vi "insert.vi"(8 "error in (no error)":errorcluster, 11 "DataCollectionDL110128Streaming in":refnum<class "DataCollectionDL110128Streaming.lvclass">) -> (0 "error out":errorcluster, 3 "DataCollectionDL110128Streaming out":refnum<class "DataCollectionDL110128Streaming.lvclass">)   [LabVIEW 2010, in "DataCollectionDL110128Streaming.lvclass"]
uses:
  DataCollectionDL110128Streaming.lvclass
  DataCollectionDL110128Streaming.lvclass/DataCollectionDL110128Streaming.ctl
  common/classes/GenericComponent/GenericComponent/class_data.vi
  common/classes/GenericComponent/GenericComponent/GenericComponent.lvclass
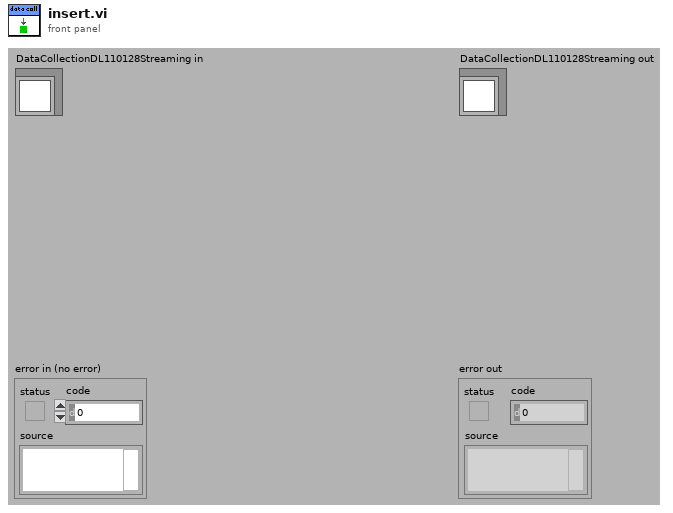
[diagram p1: front panel]
types:
  T1 = enum16{"open", "replace", "create", "open or create", "replace or create", "replace or create with confirmation"}
  T2 = typedef "pixel_raw_data_array.ctl" = dbl[][]
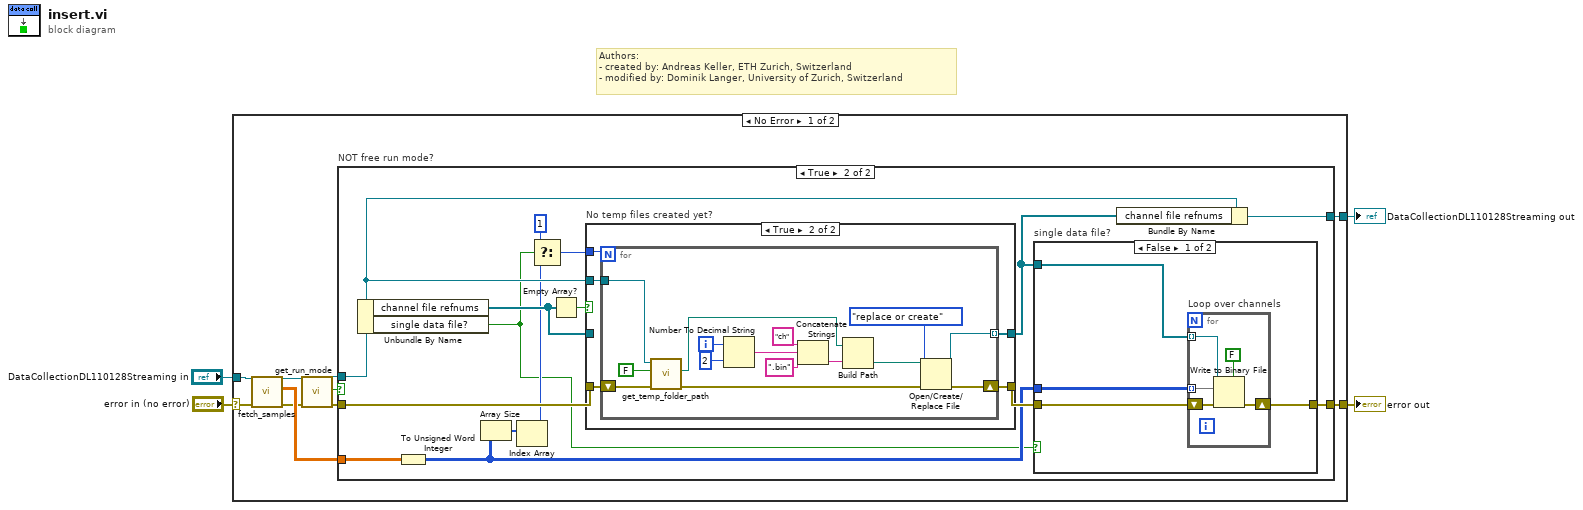
[diagram p0: block diagram]
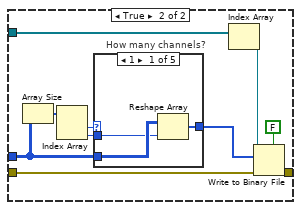
[diagram p3: hidden frame]
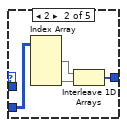
[diagram p4: hidden frame]
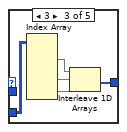
[diagram p5: hidden frame]
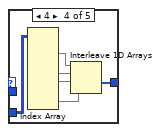
[diagram p6: hidden frame]
diagram:
  # "Authors: \n- created by: Andreas Keller, ETH Zurich, Switzerland\n- modified by: Dominik Langer, University of Zurich, Switzerland"
  n1 = case shown="No Error" "error in (no error)" {
    selector: "error in (no error)" -> [w13 w92]
    tunnel: [w12 w92] -> w3
    tunnel: [w11 w91] -> w1
    tunnel: "DataCollectionDL110128Streaming in" -> [w14 w91]
    frame No Error {
      n2 = call-dynamic "fetch_samples.vi"("error in (no error)"=w13, "GenericToplevelComponent in"=w14) -> ("error out"=w9:errorcluster, "channels raw data block"=w10:T2, "GenericToplevelComponent out"=w7:refnum<class "DataCollectionDL110128Streaming.lvclass">)  [unwired: 6 in, 1 out]
      n3 = call "get_run_mode.vi"("error in (no error)"=w9, "GenericPlugin in"=w7) -> ("error out"=w8:errorcluster, "GenericPlugin out"=w5:refnum<class "DataCollectionDL110128Streaming.lvclass">, "is NOT free run?"=w6:bool)  [unwired: 5 in, 2 out]
      n4 = case "NOT free run mode?" shown="True" w6 {
        tunnel: [w16 w29] -> w12
        tunnel: [w15 w27] -> w11
        tunnel: w10 -> [_ w23]
        tunnel: w8 -> [w16 w25]
        tunnel: w5 -> [w15 w24]
        frame False {
        }
        frame True {
          n5 = Unbundle By Name(w24) -> ("channel file refnums"=w31:refnum<file>[], "single data file?"=w17:bool)
          n6 = To Unsigned Word Integer(number=w23) -> (unsigned 16bit integer=w22:u16[][])
          n7 = Array Size(array=w22) -> (size(s)=w21:i32[])
          n8 = Index Array(array=w21) -> (element=w18:i32)  [unwired: 1 in]
          n9 = Select(t=1, s=w17, f=w18) -> (s? t:f=w20:i32)
          n10 = Empty Array?(array=w31) -> (empty?=w26:bool)
          n11 = case "No temp files created yet?" shown="True" w26 {
            tunnel: w25 -> [w70 w75]
            tunnel: [w70 w74] -> w30
            tunnel: w31 -> [w69 _]
            tunnel: [w69 w73] -> w28
            tunnel: w24 -> [_ w72]
            tunnel: w20 -> [_ w71]
            frame False {
            }
            frame True {
              n12 = for {
                N: w71 -> [_]
                shift-right: [w90] -> w74
                shift-left: w75 -> [w89]
                tunnel: [w88] -> w73 mode=indexing
                tunnel: w72 -> [w87]
                i -> [w83]
                n13 = call-dynamic "get_temp_folder_path.vi"("error in (no error)"=w89, "flush?"=FALSE, "GenericComponent in"=w87) -> ("error out"=w77:errorcluster, "temp path"=w76:path)  [unwired: 6 in, 1 out]
                n14 = Number To Decimal String(number=w83, width (-)=i16 2) -> (decimal integer string=w81:string)
                n15 = Concatenate Strings("ch", w81, ".bin") -> (w80:string)
                n16 = Build Path(base path=w76, name or relative path=w80) -> (appended path=w84:path)
                n17 = Open/Create/Replace File(file path (use dialog)=w84, error in=w77, operation (0:open)=T1."replace or create") -> (refnum out=w88:refnum<file>, error out=w90:errorcluster)  [unwired: 3 in, 1 out]
              }
            }
          }
          n18 = case "single data file?" shown="False" w17 {
            tunnel: w30 -> [w35 w47]
            tunnel: [w34 w46] -> w29
            tunnel: w28 -> [w33 w49]
            tunnel: w22 -> [w32 w41]
            frame False {
              n19 = for "Loop over channels" {
                tunnel: w33 -> [w38] mode=indexing
                tunnel: w32 -> [w36] mode=indexing
                shift-right: [w39] -> w34
                shift-left: w35 -> [w40]
                n20 = Write to Binary File(file (use dialog)=w38, data=w36, error in=w40, 5:FALSE ("prepend array or string size? (T)")) -> (error out=w39:errorcluster)  [unwired: 2 in, 2 out]
              }
            }
            frame True {
              n21 = Array Size(array=w41) -> (size(s)=w45:i32[])
              n22 = Index Array(array=w45) -> (element #1=w44:i32, element #2=w43:i32)  [unwired: 2 in]
              n23 = case "How many channels?" shown="1" w44 {
                tunnel: w41 -> [w53 w56 w60 w64 _]
                tunnel: w43 -> [w52 _ _ _ _]
                tunnel: [w51 w57 w59 w65 _] -> w42
                frame 1 {
                  n24 = Reshape Array(w53, w52) -> (w51:u16[])
                }
                frame 2 {
                  n25 = Index Array(array=w56) -> (element #1=w55:u16[], element #2=w54:u16[])  [unwired: 4 in]
                  n26 = Interleave 1D Arrays(w55, w54) -> (w57:u16[])
                }
                frame 3 {
                  n27 = Index Array(array=w60) -> (element #1=w62:u16[], element #2=w61:u16[], element #3=w58:u16[])  [unwired: 6 in]
                  n28 = Interleave 1D Arrays(w62, w61, w58) -> (w59:u16[])
                }
                frame 4 {
                  n29 = Index Array(array=w64) -> (element #1=w66:u16[], element #2=w67:u16[], element #3=w68:u16[], element #4=w63:u16[])  [unwired: 8 in]
                  n30 = Interleave 1D Arrays(w66, w67, w68, w63) -> (w65:u16[])
                }
                frame Default {
                  # "Not supported..."
                }
              }
              n31 = Index Array(array=w49) -> (element=w48:refnum<file>)  [unwired: 1 in]
              n32 = Write to Binary File(file (use dialog)=w48, data=w42, error in=w47, 5:FALSE ("prepend array or string size? (T)")) -> (error out=w46:errorcluster)  [unwired: 2 in, 2 out]
            }
          }
          n33 = Bundle By Name(cluster=w24, "channel file refnums"=w28) -> (w27:refnum<class "DataCollectionDL110128Streaming.lvclass">)
        }
      }
    }
    frame Error {
    }
  }
  "error out" <- w3
  "DataCollectionDL110128Streaming out" <- w1
